vi "BRig_RT__Case_Exp__State_endTrial__v2.vi"(6 "input_dataBlock":u16[][](array[numeric]), 9 "input_timeStamp_start":dbl, 10 "input_dataTrial":u16[][](array[numeric]), 11 "input_dataCurrent":u16[](array[numeric])) -> (0 "output_BTPRavg":dbl, 1 "output_T2Ravg":dbl, 2 "output_dataTrial":u16[][](array[numeric]), 3 "output_dataCurrent":u16[](array[numeric]), 4 "output_R(F)_or_L(T)":bool, 5 "output_runTime":dbl)   [LabVIEW 2014]
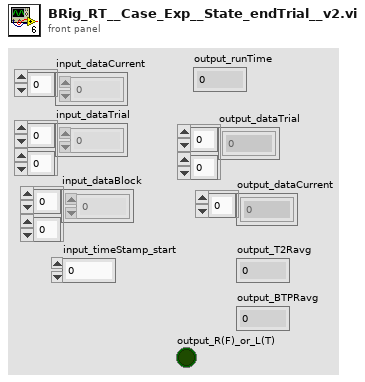
[diagram p1: front panel]
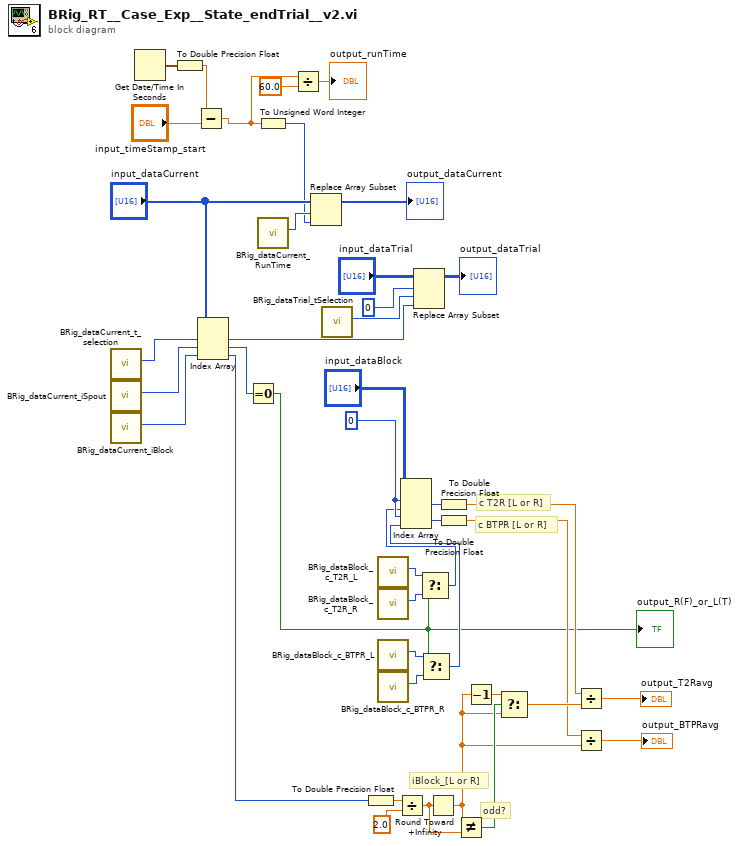
[diagram p0: block diagram]
diagram:
  w22 = 0
  # "c BTPR [L or R]"
  # "c T2R [L or R]"
  # "odd?"
  # "iBlock_[L or R]"
  n1 = call "BRig_dataCurrent_t_selection.vi"() -> ("output_t_selection"=w31:i32)  [unwired: 11 in]
  n2 = call "BRig_dataCurrent_iSpout.vi"() -> ("output_iSpout"=w26:i32)  [unwired: 11 in]
  n3 = call "BRig_dataCurrent_iBlock.vi"() -> ("output_iBlock"=w24:i32)  [unwired: 11 in]
  n4 = Get Date/Time In Seconds() -> (seconds since 1Jan1904=w37:timestamp)
  n5 = To Double Precision Float(number=w37) -> (double precision float=w35:dbl)
  n6 = Subtract(x=w35, y="input_timeStamp_start") -> (x-y=w29:dbl)
  n7 = Index Array(array="input_dataCurrent", index #1=w31, index #2=w26, index #3=w24) -> (element #1=w30:u16, element #2=w25:u16, element #3=w21:u16)
  n8 = Equal To 0?(x=w25) -> (x = 0?=w1:bool)
  "output_R(F)_or_L(T)" <- w1
  n9 = To Unsigned Word Integer(number=w29) -> (unsigned 16bit integer=w34:u16)
  n10 = call "BRig_dataCurrent_RunTime.vi"() -> ("output_RunTime"=w38:i32)  [unwired: 11 in]
  n11 = Divide(x=w29, y=60.0) -> (x/y=→"output_runTime":dbl)
  n12 = Replace Array Subset(array="input_dataCurrent", new element=w34, index=w38) -> (→"output_dataCurrent":u16[])
  n13 = call "BRig_dataTrial_tSelection.vi"() -> ("output_tSelection"=w42:i32)  [unwired: 11 in]
  n14 = To Double Precision Float(number=w21) -> (double precision float=w12:dbl)
  n15 = call "BRig_dataBlock_c_T2R_L.vi"() -> ("output_c_T2R_L"=w17:i32)  [unwired: 11 in]
  n16 = call "BRig_dataBlock_c_T2R_R.vi"() -> ("output_c_T2R_R"=w18:i32)  [unwired: 11 in]
  n17 = call "BRig_dataBlock_c_BTPR_L.vi"() -> ("output_c_BTPR_L"=w15:i32)  [unwired: 11 in]
  n18 = call "BRig_dataBlock_c_BTPR_R.vi"() -> ("output_c_BTPR_R"=w16:i32)  [unwired: 11 in]
  n19 = Divide(x=w12, y=2.0) -> (x/y=w10:dbl)
  n20 = Replace Array Subset(array="input_dataTrial", new element=w30, index (row)=0, index (col)=w42) -> (→"output_dataTrial":u16[][])
  n21 = Select(t=w17, s=w1, f=w18) -> (s? t:f=w14:i32)
  n22 = Select(t=w15, s=w1, f=w16) -> (s? t:f=w13:i32)
  n23 = Index Array(array="input_dataBlock", index (row) #1=w22, index (col) #1=w14, index (row) #2=w22, index (col) #2=w13) -> (element #1=w5:u16, element #2=w6:u16)
  n24 = Round Toward +Infinity(x=w10) -> (ceil(x): smallest int >= x=w4:dbl)
  n25 = To Double Precision Float(number=w5) -> (double precision float=w3:dbl)
  n26 = To Double Precision Float(number=w6) -> (double precision float=w2:dbl)
  n27 = Not Equal?(x=w4, y=w10) -> (x != y?=w8:bool)
  n28 = Decrement(x=w4) -> (x-1=w9:dbl)
  n29 = Select(t=w9, s=w8, f=w4) -> (s? t:f=w7:dbl)
  n30 = Divide(x=w3, y=w7) -> (x/y=→"output_T2Ravg":dbl)
  n31 = Divide(x=w2, y=w4) -> (x/y=→"output_BTPRavg":dbl)
